vi "XBox Demo Client.vi"() -> ()   [LabVIEW 2015]
uses:
  XBox-Globals.vi
panel:
  in  "Vibrate":bool
  in  "Max Velocity X":dbl=2.0
  in  "Max Velocity Y":dbl=0.5
  out "Waveform Graph":dbl[](graph)
  out "A":bool
  in  "Quit":bool
  out "Y":bool
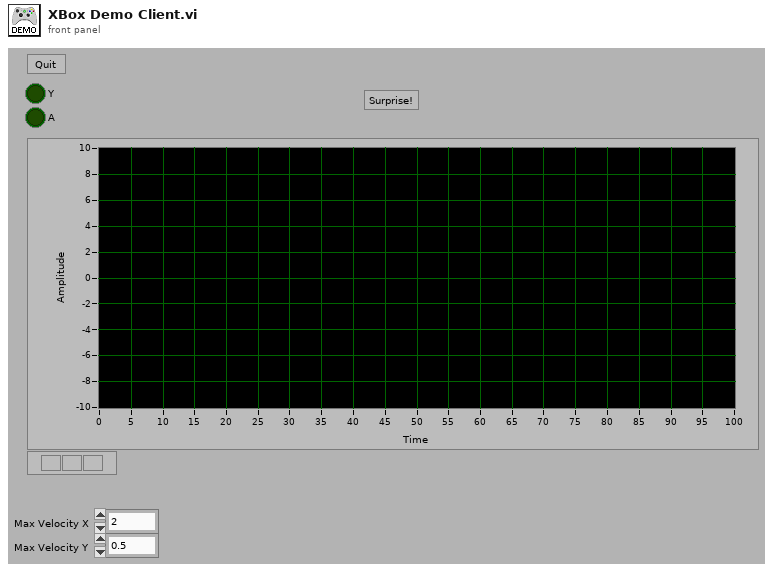
[diagram p1: front panel]
types:
  T1 = typedef "XBox-Events Ref.ctl" = refnum<event-registration>
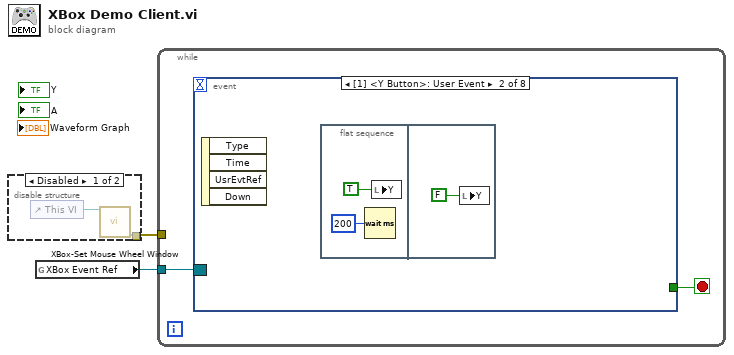
[diagram p0: block diagram]
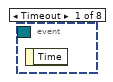
[diagram p3: hidden frame]
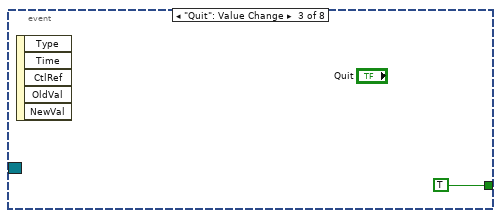
[diagram p4: hidden frame]
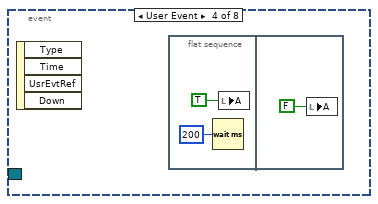
[diagram p5: hidden frame]
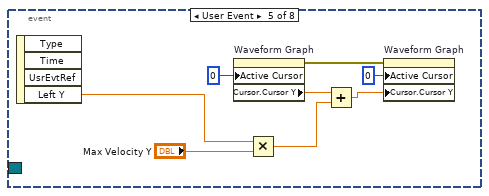
[diagram p6: hidden frame]
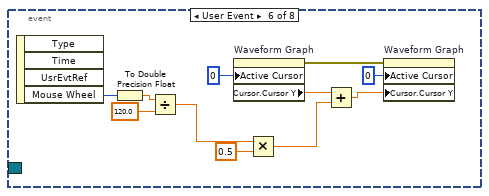
[diagram p7: hidden frame]
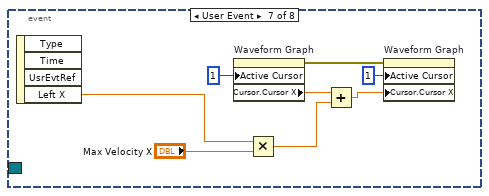
[diagram p8: hidden frame]
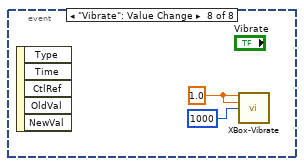
[diagram p9: hidden frame]
diagram:
  n1 = disable-structure shown="Disabled" {
    disable-tunnel: [w4 _] -> w1
    frame Disabled {
      n2 = control-ref of="This VI"() -> (w3:refnum<vi>)
      n3 = call "XBox-Set Mouse Wheel Window.vi"("VI ref"=w3) -> ("error out"=w4:errorcluster)  [unwired: 13 in, 1 out]
    }
    frame Enabled {
    }
  }
  n4 = global read "XBox-Globals.vi" "XBox Event Ref"() -> (w2:T1)
  n5 = while {
    tunnel: w2 -> [w5]
    tunnel: w1 -> [_]
    stop <- w6 stop-if-true
    n6 = event shown="[1] <Y Button>: User Event" {
      selector: w5 -> [_ _ _ _ _ _ _ _]
      dyn-events: _ -> [_ _ _ _ _ _ _ _]
      timeout: _ -> [_ _ _ _ _ _ _ _]
      tunnel: [_ _ TRUE _ _ _ _ _] -> w6
      event Timeout {
        n7 = event-data() -> ()  [unwired: 1 in, 1 out]
      }
      event User Event {
        n8 = event-data() -> ()  [unwired: 1 in, 4 out]
        n9 = flat-sequence {
          frame #0 {
            n10 = Wait (ms)(milliseconds to wait=u32 200) -> ()  [unwired: 1 out]
            n11 = local write "Y"(TRUE ("Y")) -> ()
          }
          frame #1 {
            n12 = local write "Y"(FALSE ("Y")) -> ()
          }
        }
      }
      event "Quit": Value Change {
        n13 = event-data() -> ()  [unwired: 1 in, 5 out]
      }
      event User Event {
        n14 = event-data() -> ()  [unwired: 1 in, 4 out]
        n15 = flat-sequence {
          frame #0 {
            n16 = Wait (ms)(milliseconds to wait=u32 200) -> ()  [unwired: 1 out]
            n17 = local write "A"(TRUE ("Y")) -> ()
          }
          frame #1 {
            n18 = local write "A"(FALSE ("Y")) -> ()
          }
        }
      }
      event User Event {
        n19 = event-data() -> ("Left Y"=w21:dbl)  [unwired: 1 in, 3 out]
        n20 = property on="Waveform Graph" class="WFGraph (strict)"("Active Cursor"=0 ("Cursor.Cursor Index")) -> (error out=w16:errorcluster, "Cursor.Cursor Y"=w20:dbl)  [unwired: 2 in, 1 out]
        n21 = Multiply(x=w21, y="Max Velocity Y") -> (x*y=w19:dbl)
        n22 = Add(x=w20, y=w19) -> (x+y=w15:dbl)
        n23 = property on="Waveform Graph" class="WFGraph (strict)"(error in=w16, "Active Cursor"=u32 0, "Cursor.Cursor Y"=w15) -> ()  [unwired: 1 in, 2 out]
      }
      event User Event {
        n24 = event-data() -> ("Mouse Wheel"=w25:i32)  [unwired: 1 in, 3 out]
        n25 = To Double Precision Float(number=w25) -> (double precision float=w26:dbl)
        n26 = Divide(x=w26, y=120.0) -> (x/y=w23:dbl)
        n27 = property on="Waveform Graph" class="WFGraph (strict)"("Active Cursor"=0 ("Cursor.Cursor Index")) -> (error out=w29:errorcluster, "Cursor.Cursor Y"=w32:dbl)  [unwired: 2 in, 1 out]
        n28 = Multiply(x=w23, y=0.5) -> (x*y=w31:dbl)
        n29 = Add(x=w32, y=w31) -> (x+y=w28:dbl)
        n30 = property on="Waveform Graph" class="WFGraph (strict)"(error in=w29, "Active Cursor"=u32 0, "Cursor.Cursor Y"=w28) -> ()  [unwired: 1 in, 2 out]
      }
      event User Event {
        n31 = event-data() -> ("Left X"=w40:dbl)  [unwired: 1 in, 3 out]
        n32 = property on="Waveform Graph" class="WFGraph (strict)"("Active Cursor"=1 ("Cursor.Cursor Index")) -> (error out=w35:errorcluster, "Cursor.Cursor X"=w39:dbl)  [unwired: 2 in, 1 out]
        n33 = Multiply(x=w40, y="Max Velocity X") -> (x*y=w38:dbl)
        n34 = Add(x=w39, y=w38) -> (x+y=w34:dbl)
        n35 = property on="Waveform Graph" class="WFGraph (strict)"(error in=w35, "Active Cursor"=u32 1, "Cursor.Cursor X"=w34) -> ()  [unwired: 1 in, 2 out]
      }
      event "Vibrate": Value Change {
        w42 = 1.0 ("Left Motor")
        n36 = event-data() -> ()  [unwired: 1 in, 5 out]
        n37 = call "XBox-Vibrate.vi"("Left Motor"=w42, "Right Motor"=w42, "Duration (ms)"=u32 1000) -> ()  [unwired: 12 in, 1 out]
      }
    }
  }
